vi "ooptest.vi"() -> ()   [LabVIEW 2013]
uses:
  OOP/Report.lvclass
  OOP/Test.lvclass
panel:
  in  "error in (no error)":errorcluster caption="Fehler (Eingang, kein Fehler)"
  out "error out":errorcluster caption="Fehler (Ausgang)"
  in  "Tname":string
  out "Report (Ausgang)":refnum<class "Report.lvclass">
  out "XML-String":string
  in  "Test.lvclass":refnum<class "Test.lvclass">
  in  "Report.lvclass":refnum<class "Report.lvclass">
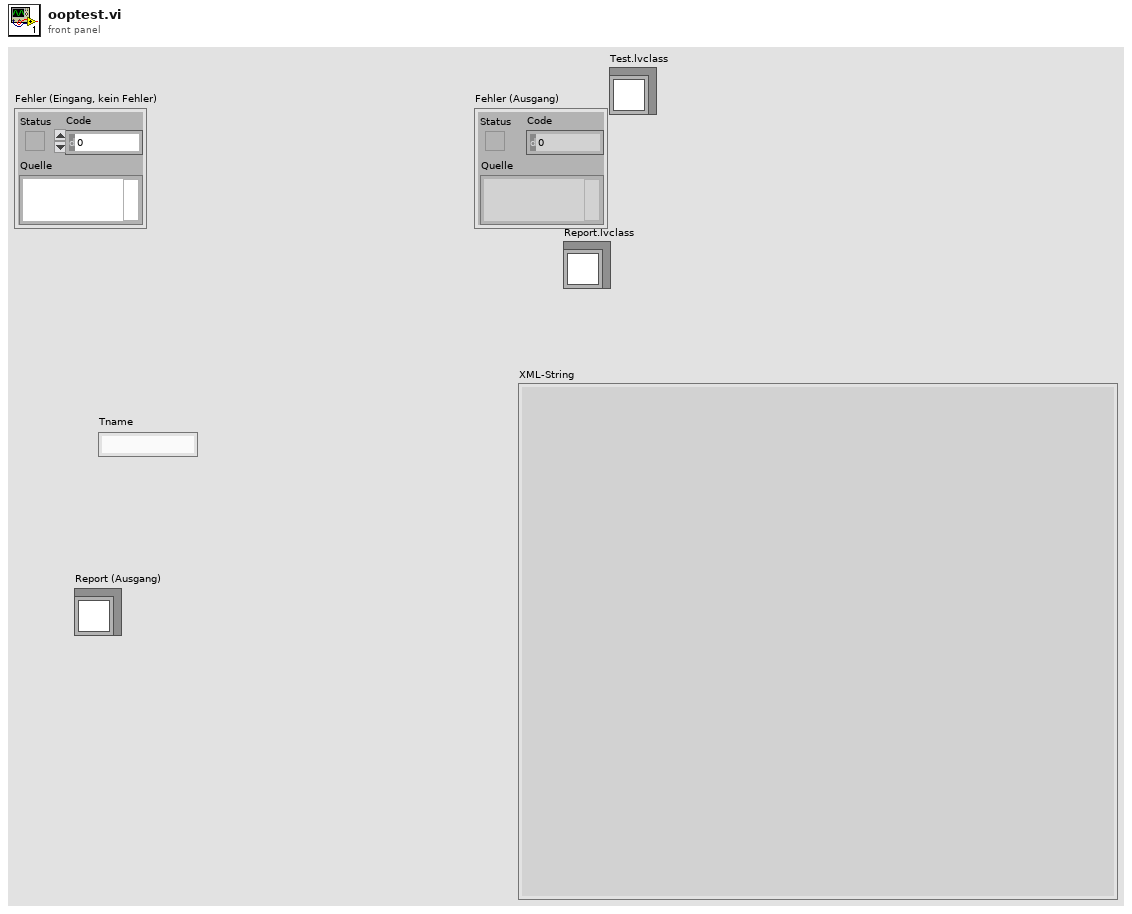
[diagram p1: front panel]
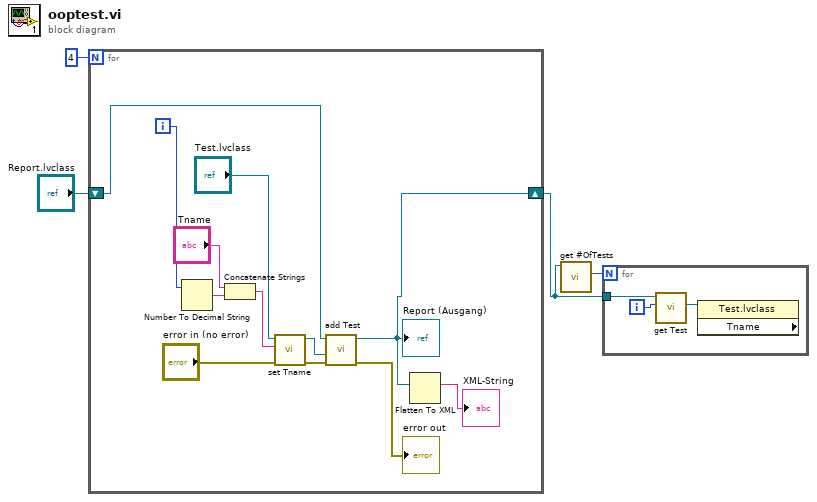
[diagram p0: block diagram]
diagram:
  n1 = for {
    N: 4 -> [_]
    shift-right: [w6] -> w1
    shift-left: "Report.lvclass" -> [w5]
    i -> [w12]
    n2 = Number To Decimal String(number=w12) -> (decimal integer string=w11:string)  [unwired: 1 in]
    n3 = Concatenate Strings("Tname", w11) -> (w10:string)
    n4 = call-dynamic "set Tname.vi"("error in (no error)"="error in (no error)", "name"=w10, "Test (Eingang)"="Test.lvclass") -> ("error out"=w14:errorcluster, "Test (Ausgang)"=w15:refnum<class "Test.lvclass">)  [unwired: 7 in]
    n5 = call-dynamic "add Test.vi"("error in (no error)"=w14, "Test.lvclass"=w15, "Report (Eingang)"=w5) -> ("error out"=→"error out":errorcluster, "Report (Ausgang)"=w6:refnum<class "Report.lvclass">)  [unwired: 7 in]
    "Report (Ausgang)" <- w6
    n6 = Flatten To XML(anything=w6) -> (xml string=→"XML-String":string)
  }
  n7 = call-dynamic "get #OfTests.vi"("Report (Eingang)"=w1) -> ("#OfTests"=w4:u32)  [unwired: 8 in, 2 out]
  n8 = for {
    N: w4 -> [_]
    tunnel: w1 -> [w19]
    i -> [w18]
    n9 = call-dynamic "get Test.vi"("index"=w18, "Report (Eingang)"=w19) -> ("Test.lvclass"=w17:refnum<class "Test.lvclass">)  [unwired: 7 in, 2 out]
    n10 = property class="Test.lvclass" props=["Tname"](reference=w17) -> ()  [unwired: 1 in, 3 out]
  }
